vi "DrivePath.vi"(2 "Parameter String":string, 3 "Reinit":bool) -> (0 "Path Follower Error":errorcluster, 1 "Increment":bool)   [LabVIEW 2023]
doc: "A mixed pursuit + feed-forward path-following algorithm configured for a swerve drive. Feed-forward and feed-back controllers are combined to produce unitless drive commands. This VI is designed to integrated with the FRC 4265 Autonomous Path Planner. The Search Window can be specified in seconds - longer search windows are more robust to recovering from large deviations from the path but may cause the robot to \"jump\" ahead when following tight loops or turns. The Look-Ahead Time specifies the furthest ahead the pursuit point can be. Supports selecting different paths based on the alliance color.\n\nParameters:\n1. acceptable distance error --> (in) [0,614.25]\n2. acceptable angle error --> (deg) [0,180]\n3. path follow timeout --> (ms) [0,15000] set to -1 for no timeout\n3. name of the autonomous path\n4. specifiy whether or not the robot can add a suffix to the selected path name {normal,robot_suffix}"
uses:
  5c80b45a-8b82-4ca3-a7a6-7ac929992d21.vi
  SafeParser_Float.vi
  SafeParser_Integer.vi
  SafeParser_String.vi
  GlobalPoseAndTargeting.vi
  GlobalAutonomous.vi
  GlobalDriverStationCommands.vi
panel:
  out "PID Strafe":T1(graph)
  in  "PID Tuning Strafe":T2={"Kp"=0.008, "Ki"=0.0, "Kd"=0.0, "N-Diff"=5, "N-Int"=10, "Int Error Window"=20.0, "Max Ouput"=1.0, "Min Output"=-1.0} {"Int Error Window" min=0.0; "N-Int" min=2; "N-Diff" min=2; "Kd" min=0.0; "Ki" min=0.0; "Kp" min=0.0}
  out "PID Heading":T1(graph)
  in  "PID Tuning Heading":T2={"Kp"=0.0035, "Ki"=0.003, "Kd"=0.0, "N-Diff"=10, "N-Int"=10, "Int Error Window"=10.0, "Max Ouput"=0.5, "Min Output"=-0.5} {"Int Error Window" min=0.0; "N-Int" min=2; "N-Diff" min=2; "Kd" min=0.0; "Ki" min=0.0; "Kp" min=0.0}
  out "Path and Robot Pose":cluster{dbl[], dbl[]}[](graph)
  in  "Plot":bool
  in  "Max Look-Ahead Time (s)":dbl=0.25
  in  "Search Window (s)":dbl=0.25
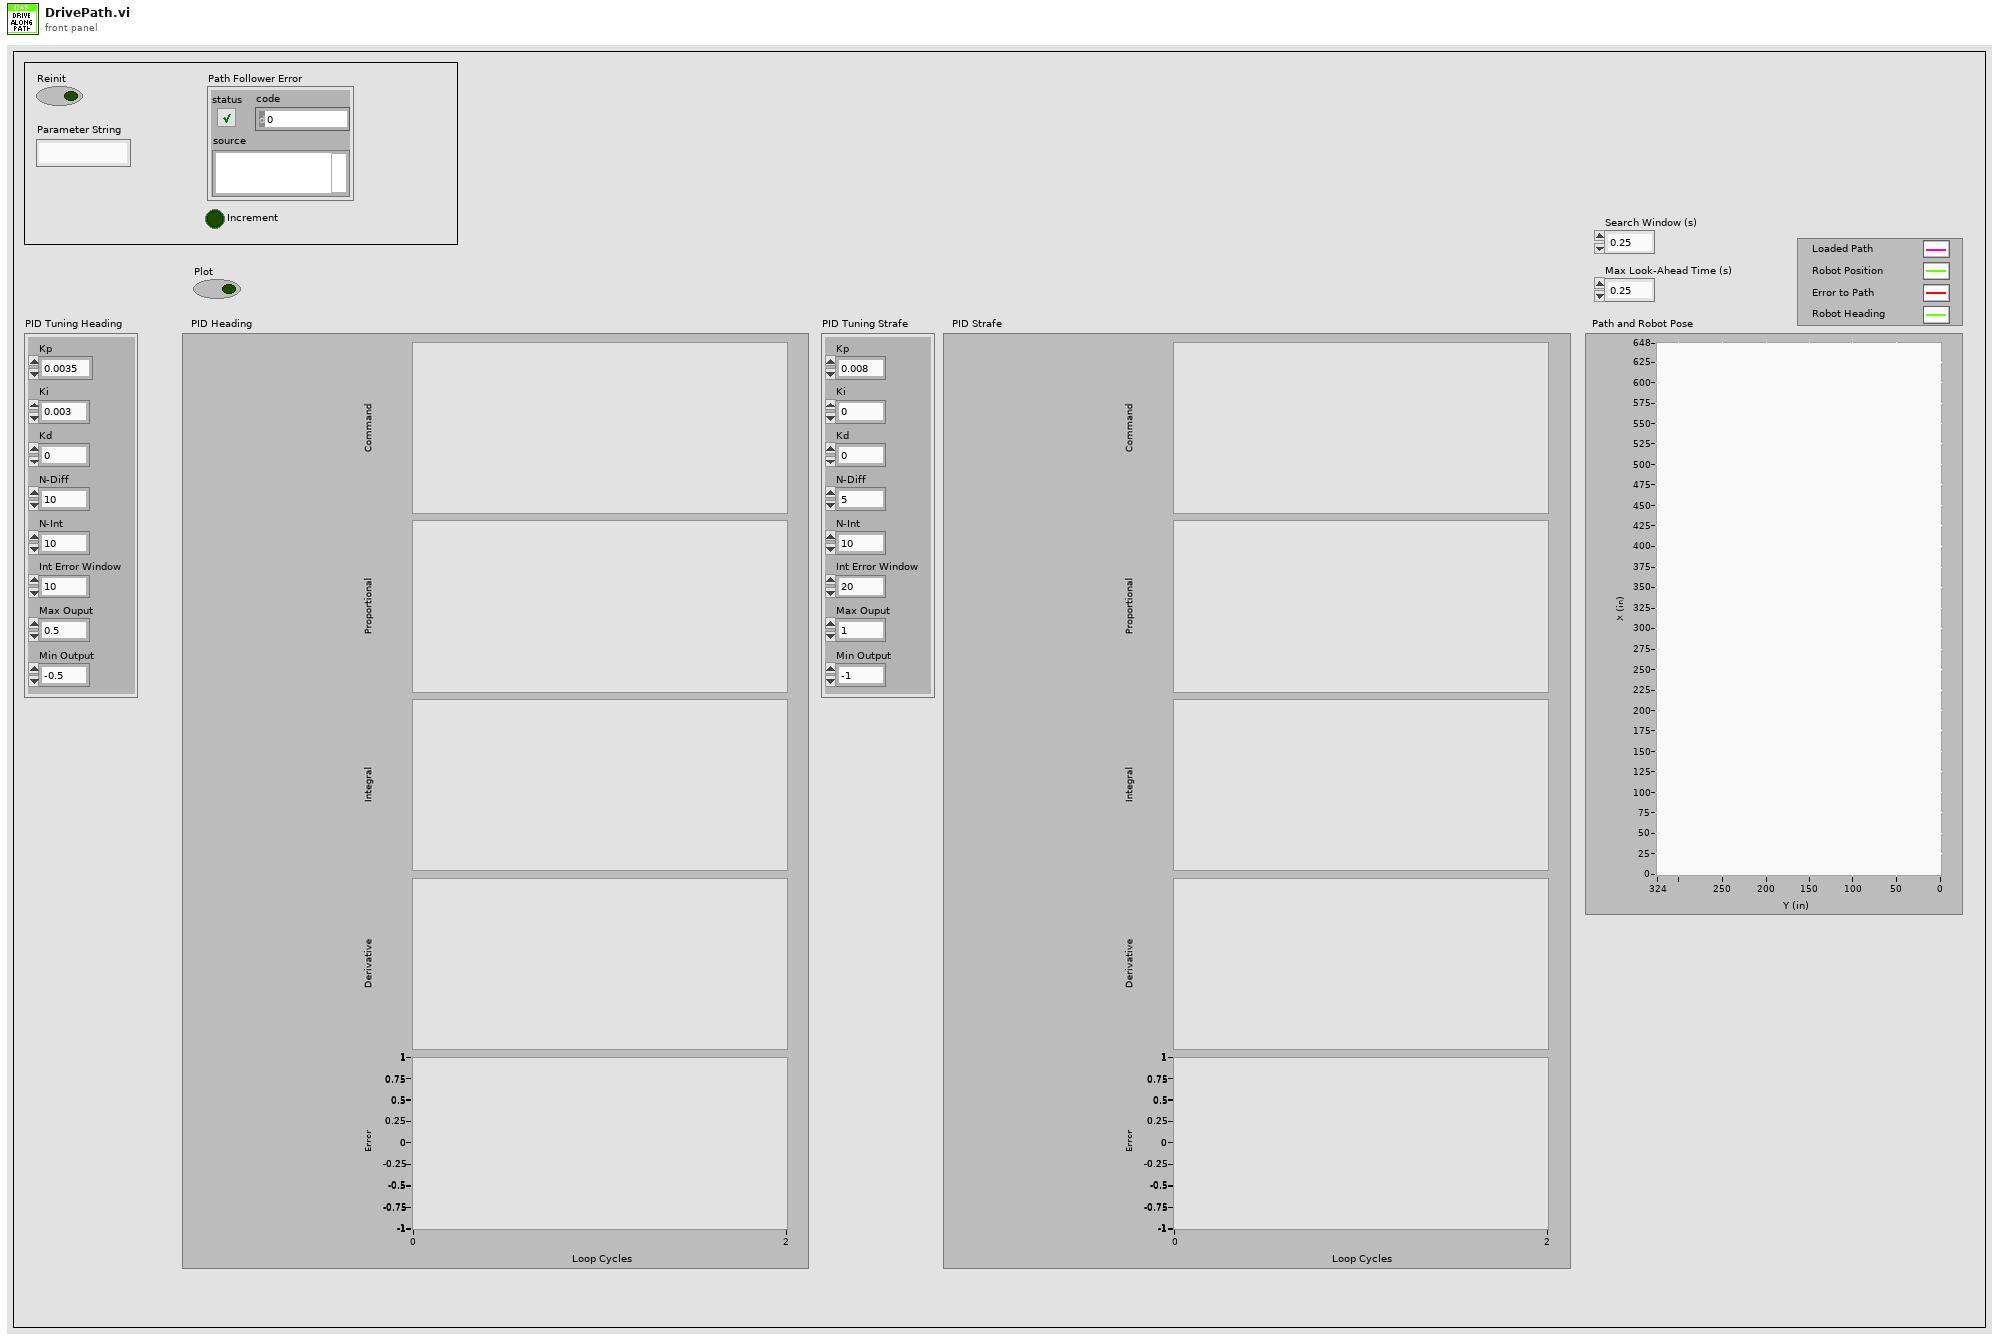
[diagram p1: front panel]
types:
  T1 = cluster{"Command":dbl, "Proportional":dbl, "Integral":dbl, "Derivative":dbl, "Goal":dbl}
  T2 = cluster{"Kp":dbl, "Ki":dbl, "Kd":dbl, "N-Diff":i32, "N-Int":i32, "Int Error Window":dbl, "Max Ouput":dbl, "Min Output":dbl}
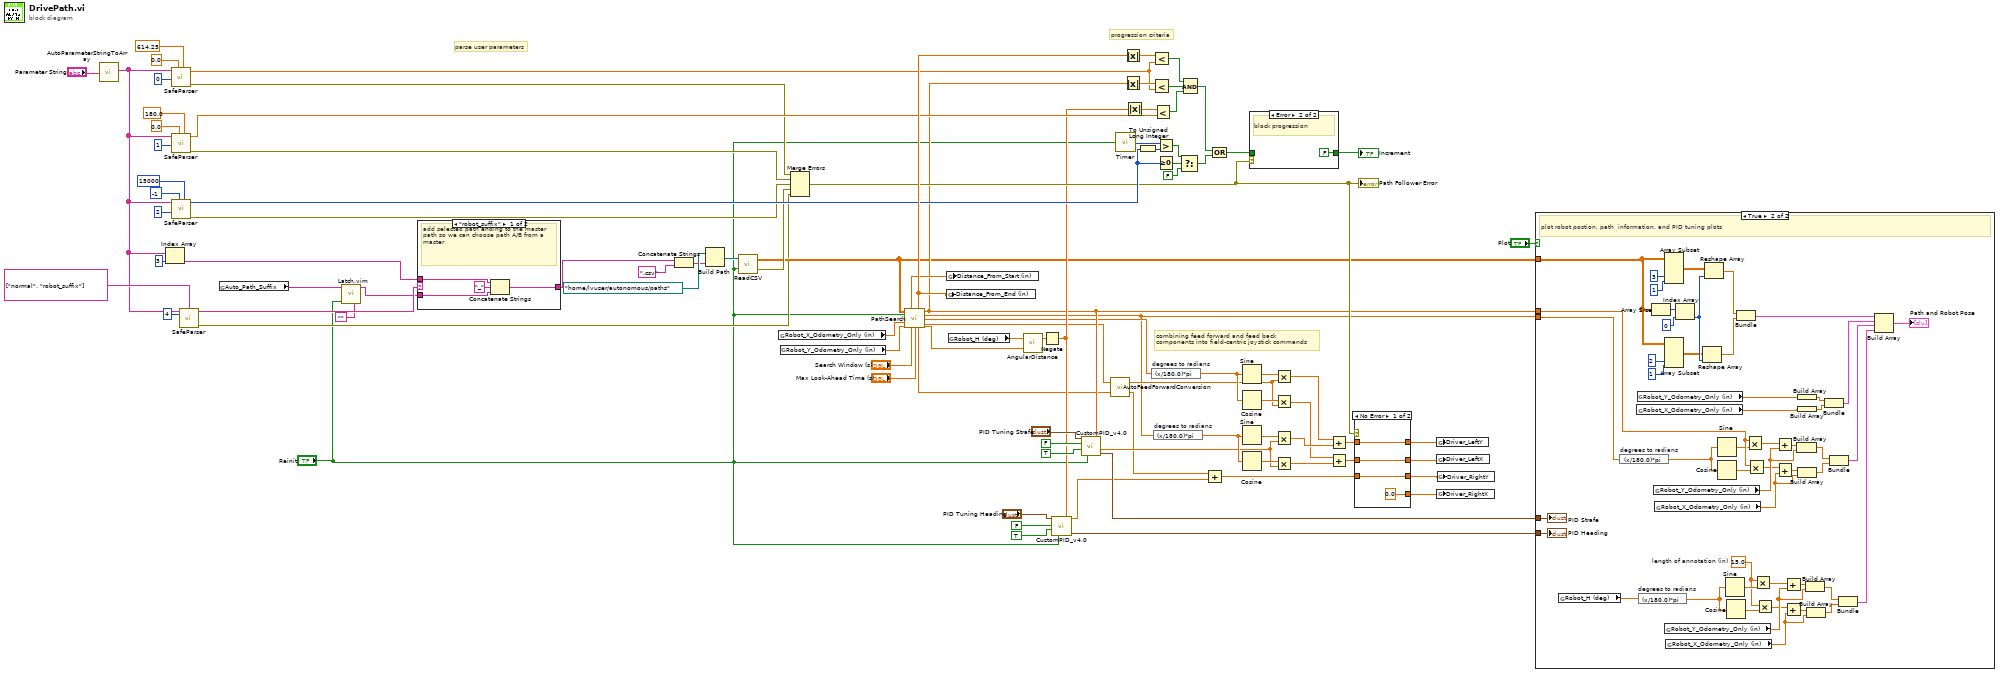
[diagram p0: block diagram]
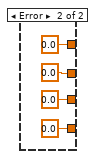
[diagram p5: hidden frame]
diagram:
  # "parse user parameters"
  # "progression criteria"
  # "combining feed forward and feed back\ncomponents into field-centric joystick commands"
  n1 = call "AutoParameterStringToArray.vi"("Parameter String"="Parameter String") -> ("Parsed Parameters"=w25:string[])
  n2 = Index Array(array=w25, index=3) -> (element=w28:string)
  n3 = call-poly "SafeParser.vi"("Maximum"=614.25, "Minimum"=0.0, "Array Index"=0 ("Parameter Index"), "String Array"=w25) -> ("Error Out"=w57:errorcluster, "Typecast  Value"=w65:dbl)  [unwired: 6 in]
  n4 = call-poly "SafeParser.vi"("Maximum"=180.0, "Minimum"=0.0, "Array Index"=1 ("Parameter Index"), "String Array"=w25) -> ("Error Out"=w58:errorcluster, "Typecast  Value"=w62:dbl)  [unwired: 6 in]
  n5 = call-poly "SafeParser.vi"("Maximum"=15000, "Minimum"=-1, "Array Index"=2 ("Parameter Index"), "String Array"=w25) -> ("Error Out"=w59:errorcluster, "Typecast  Value"=w70:i32)  [unwired: 6 in]
  n6 = call-poly "SafeParser.vi"("Allowed Values"=string[] ["normal", "robot_suffix"], "Array Index"=4, "String Array"=w25) -> ("Error Out"=w24:errorcluster, "Typecast Value"=w26:string)  [unwired: 7 in]
  n7 = global read "GlobalAutonomous.vi" "Auto_Path_Suffix"() -> (w10:string)
  n8 = call "Latch.vim"("Default Value"="", "Latch Signal"="Reinit", "Latch Value"=w10) -> ("Latched"=w7:string)  [unwired: 8 in]
  n9 = case shown="\"robot_suffix\"" w26 {
    tunnel: w28 -> [w99 w100]
    tunnel: [w98 w100] -> w27
    tunnel: w7 -> [w97 _]
    frame "robot_suffix" {
      # "add selected path ending to the master \npath so we can choose path A/B from a master"
      n10 = Concatenate Strings(w99, "_" ("string"), w97) -> (w98:string)
    }
    frame "normal", Default {
    }
  }
  n11 = Concatenate Strings(w27, ".csv" ("string")) -> (w89:string)
  n12 = Build Path(base path=path "/home/lvuser/autonomous/paths" ("path"), name or relative path=w89) -> (appended path=w94:path)
  n13 = call "ReadCSV.vi"("Reinit"="Reinit", "File Path (.csv)"=w94) -> ("File Open Eror"=w60:errorcluster, "Data (index by row)"=w33:dbl[][])
  n14 = global read "GlobalPoseAndTargeting.vi" "Robot_X_Odometry_Only (in)"() -> (w93:dbl)
  n15 = global read "GlobalPoseAndTargeting.vi" "Robot_Y_Odometry_Only (in)"() -> (w92:dbl)
  n16 = Merge Errors(w57, w58, w59, w60, w24) -> (w61:errorcluster)
  "Path Follower Error" <- w61
  n17 = call "PathSearch.vi"("Path"=w33, "Reint"="Reinit", "Robot X (in)"=w93, "Robot Y (in)"=w92, "Search Window (s)"="Search Window (s)", "Look-Ahead Time (s)"="Max Look-Ahead Time (s)") -> ("Distance from Start (in)"=w83:dbl, "Distance from End (in)"=w84:dbl, "Feed Back Distance Error (in)"=w39:dbl, "Feed Back Pointing Angle (deg)"=w18:dbl, "Feed Forward Pointing Angle (deg)"=w23:dbl, "Feed Forward Velocity (in/s)"=w5:dbl, "Feed Forward Rotational Velocity (deg/s)"=w4:dbl, "Robot Heading Goal (deg)"=w73:dbl)  [unwired: 2 in]
  n18 = global write "GlobalAutonomous.vi" "Distance_From_End (in)"(w84) -> ()
  n19 = global write "GlobalAutonomous.vi" "Distance_From_Start (in)"(w83) -> ()
  n20 = global read "GlobalPoseAndTargeting.vi" "Robot_H (deg)"() -> (w46:dbl)
  n21 = call "AngularDistance.vi"("Goal Angle (deg) [0,360]"=w73, "Current Angle (deg) [-Inf,+Inf]"=w46) -> ("Signed Angular Distance (deg) [-180,+180]"=w44:dbl)  [unwired: 1 out]
  n22 = Negate(x=w44) -> (-x=w43:dbl)
  n23 = call "CustomPID_v4.0.vi"("PID Tuning Parameters"="PID Tuning Heading", "Custom Error Calculation"=w43, "Reset on Goal Change ?"=FALSE, "Use Custom Error Calculation ?"=TRUE, "Reinit"="Reinit") -> ("Command"=w3:dbl, "Controller Summary"=w42:T1)  [unwired: 7 in, 2 out]
  n24 = call "CustomPID_v4.0.vi"("PID Tuning Parameters"="PID Tuning Strafe", "Custom Error Calculation"=w39, "Reset on Goal Change ?"=FALSE, "Use Custom Error Calculation ?"=TRUE, "Reinit"="Reinit") -> ("Command"=w17:dbl, "Controller Summary"=w49:T1)  [unwired: 7 in, 2 out]
  n25 = call "AutoFeedForwardConversion.vi"("Planned Rotational Velocity (deg/s)"=w4, "Planned Ground Velocity (in/s)"=w5) -> ("Equivalent Rotation Joystick Command (ul)"=w1:dbl, "Equivalent Strafe Joystick Command (ul)"=w22:dbl)
  n26 = call "Timer.vi"("Reset Timer"="Reinit") -> ("Time (ms)"=w74:u32)
  n27 = Absolute Value(x=w84) -> (abs(x)=w75:dbl)
  n28 = Absolute Value(x=w39) -> (abs(x)=w76:dbl)
  n29 = Absolute Value(x=w43) -> (abs(x)=w82:dbl)
  n30 = To Unsigned Long Integer(number=w70) -> (unsigned 32bit integer=w80:u32)
  n31 = expression code="(x/180.0)*pi" "degrees to radians"(w23) -> (w87:dbl)
  n32 = Less?(x=w75, y=w65) -> (x < y?=w36:bool)
  n33 = Less?(x=w76, y=w65) -> (x < y?=w37:bool)
  n34 = Less?(x=w82, y=w62) -> (x < y?=w38:bool)
  n35 = expression code="(x/180.0)*pi" "degrees to radians"(w18) -> (w21:dbl)
  n36 = Greater?(x=w74, y=w80) -> (0:w78:bool)
  n37 = Greater Or Equal To 0?(x=w70) -> (x >= 0?=w79:bool)
  n38 = Select(t=w78, s=w79, f=FALSE) -> (s? t:f=w34:bool)
  n39 = Compound Arithmetic op=AND(w36, w37, w38) -> (w35:bool)
  n40 = Add(x=w1, y=w3) -> (x+y=w2:dbl)
  n41 = Compound Arithmetic op=OR(w35, w34) -> (w81:bool)
  n42 = Sine(x=w87) -> (sin(x)=w86:dbl)
  n43 = Cosine(x=w87) -> (cos(x)=w85:dbl)
  n44 = Sine(x=w21) -> (sin(x)=w20:dbl)
  n45 = Cosine(x=w21) -> (cos(x)=w19:dbl)
  n46 = case shown="Error" w61 {
    tunnel: [w101 FALSE] -> w6
    tunnel: w81 -> [w101 _]
    frame No Error {
      # "allow progression"
    }
    frame Error {
      # "block progression"
    }
  }
  "Increment" <- w6
  n47 = Multiply(x=w86, y=w22) -> (x*y=w16:dbl)
  n48 = Multiply(x=w85, y=w22) -> (x*y=w14:dbl)
  n49 = Multiply(x=w20, y=w17) -> (x*y=w15:dbl)
  n50 = Multiply(x=w19, y=w17) -> (x*y=w13:dbl)
  n51 = Add(x=w16, y=w15) -> (x+y=w12:dbl)
  n52 = Add(x=w14, y=w13) -> (x+y=w11:dbl)
  n53 = case shown="No Error" w61 {
    tunnel: [w103 0.0] -> w41
    tunnel: [w106 0.0 ("upper limit")] -> w88
    tunnel: [w104 0.0] -> w40
    tunnel: w2 -> [w106 _]
    tunnel: [0.0 0.0] -> w45
    tunnel: w12 -> [w104 _]
    tunnel: w11 -> [w103 _]
    frame No Error {
    }
    frame Error {
    }
  }
  n54 = global write "GlobalDriverStationCommands.vi" "Driver_LeftY"(w40) -> ()
  n55 = global write "GlobalDriverStationCommands.vi" "Driver_LeftX"(w41) -> ()
  n56 = global write "GlobalDriverStationCommands.vi" "Driver_RightX"(w45) -> ()
  n57 = global write "GlobalDriverStationCommands.vi" "Driver_RightY"(w88) -> ()
  n58 = case shown="True" "Plot" {
    tunnel: w18 -> [_ w154]
    tunnel: w49 -> [_ w153]
    tunnel: w42 -> [_ w152]
    tunnel: w39 -> [_ w151]
    tunnel: w33 -> [_ w150]
    frame False {
    }
    frame True {
      w115 = 15.0  # length of annotation (in)
      # "plot robot postion, path  information, and PID tuning plots"
      n59 = global read "GlobalPoseAndTargeting.vi" "Robot_H (deg)"() -> (w155:dbl)
      n60 = expression code="(x/180.0)*pi" "degrees to radians"(w154) -> (w127:dbl)
      n61 = global read "GlobalPoseAndTargeting.vi" "Robot_X_Odometry_Only (in)"() -> (w158:dbl)
      n62 = global read "GlobalPoseAndTargeting.vi" "Robot_Y_Odometry_Only (in)"() -> (w159:dbl)
      n63 = expression code="(x/180.0)*pi" "degrees to radians"(w155) -> (w116:dbl)
      n64 = Array Size(array=w150) -> (size(s)=w146:i32[])
      n65 = global read "GlobalPoseAndTargeting.vi" "Robot_Y_Odometry_Only (in)"() -> (w137:dbl)
      n66 = global read "GlobalPoseAndTargeting.vi" "Robot_X_Odometry_Only (in)"() -> (w136:dbl)
      n67 = Array Subset(array=w150, index (col)=2 ("index"), length (col)=1 ("length")) -> (w144:dbl[][])  [unwired: 2 in]
      n68 = Array Subset(array=w150, index (col)=3 ("index"), length (col)=1 ("length")) -> (w145:dbl[][])  [unwired: 2 in]
      n69 = global read "GlobalPoseAndTargeting.vi" "Robot_Y_Odometry_Only (in)"() -> (w126:dbl)
      n70 = global read "GlobalPoseAndTargeting.vi" "Robot_X_Odometry_Only (in)"() -> (w125:dbl)
      n71 = Index Array(array=w146, index=0) -> (element=w147:i32)
      n72 = Reshape Array(w144, w147) -> (w112:dbl[])
      n73 = Reshape Array(w145, w147) -> (w113:dbl[])
      n74 = Sine(x=w127) -> (sin(x)=w128:dbl)
      n75 = Cosine(x=w127) -> (cos(x)=w129:dbl)
      n76 = Sine(x=w116) -> (sin(x)=w117:dbl)
      n77 = Cosine(x=w116) -> (cos(x)=w118:dbl)
      n78 = Bundle(w113, w112) -> (w149:cluster{dbl[], dbl[]})  [unwired: 1 in]
      n79 = Multiply(x=w151, y=w128) -> (x*y=w130:dbl)
      n80 = Multiply(x=w151, y=w129) -> (x*y=w131:dbl)
      n81 = Multiply(x=w115, y=w117) -> (x*y=w119:dbl)
      n82 = Multiply(x=w115, y=w118) -> (x*y=w120:dbl)
      n83 = Add(x=w130, y=w137) -> (x+y=w132:dbl)
      n84 = Add(x=w131, y=w136) -> (x+y=w133:dbl)
      n85 = Add(x=w119, y=w126) -> (x+y=w121:dbl)
      n86 = Add(x=w120, y=w125) -> (x+y=w122:dbl)
      n87 = Build Array(w132, w137) -> (w134:dbl[])
      n88 = Build Array(w159) -> (w156:dbl[])
      n89 = Build Array(w158) -> (w157:dbl[])
      n90 = Build Array(w133, w136) -> (w135:dbl[])
      n91 = Build Array(w121, w126) -> (w123:dbl[])
      n92 = Build Array(w122, w125) -> (w124:dbl[])
      n93 = Bundle(w156, w157) -> (w138:cluster{dbl[], dbl[]})  [unwired: 1 in]
      n94 = Bundle(w134, w135) -> (w114:cluster{dbl[], dbl[]})  [unwired: 1 in]
      n95 = Bundle(w123, w124) -> (w111:cluster{dbl[], dbl[]})  [unwired: 1 in]
      n96 = Build Array(w149, w138, w114, w111) -> (→"Path and Robot Pose":cluster{dbl[], dbl[]}[])
      "PID Strafe" <- w153
      "PID Heading" <- w152
    }
  }
